vi "VisionLab_LHFind_Main.vi"() -> ()   [LabVIEW 2014]
uses:
  <vilib>/vision/Image Controls.llb/IMAQ Image.ctl
  <vilib>/userdefined/High Color/IMAQdx.ctl
  <vilib>/vision/driver/NI_Vision_Acquisition_Software.lvlib
panel:
  out "LH_Find":T1
  out "servo error out":errorcluster
  in  "Destination Point":cluster{"DestinationX":dbl, "DestinationY":dbl}={"DestinationX"=520.0, "DestinationY"=320.0}
  out "error out":errorcluster
  out "Live Input":T1(plugin-control)
  out "Running":bool
  in  "stop":bool
  out "FindLaser Out":T1(plugin-control)
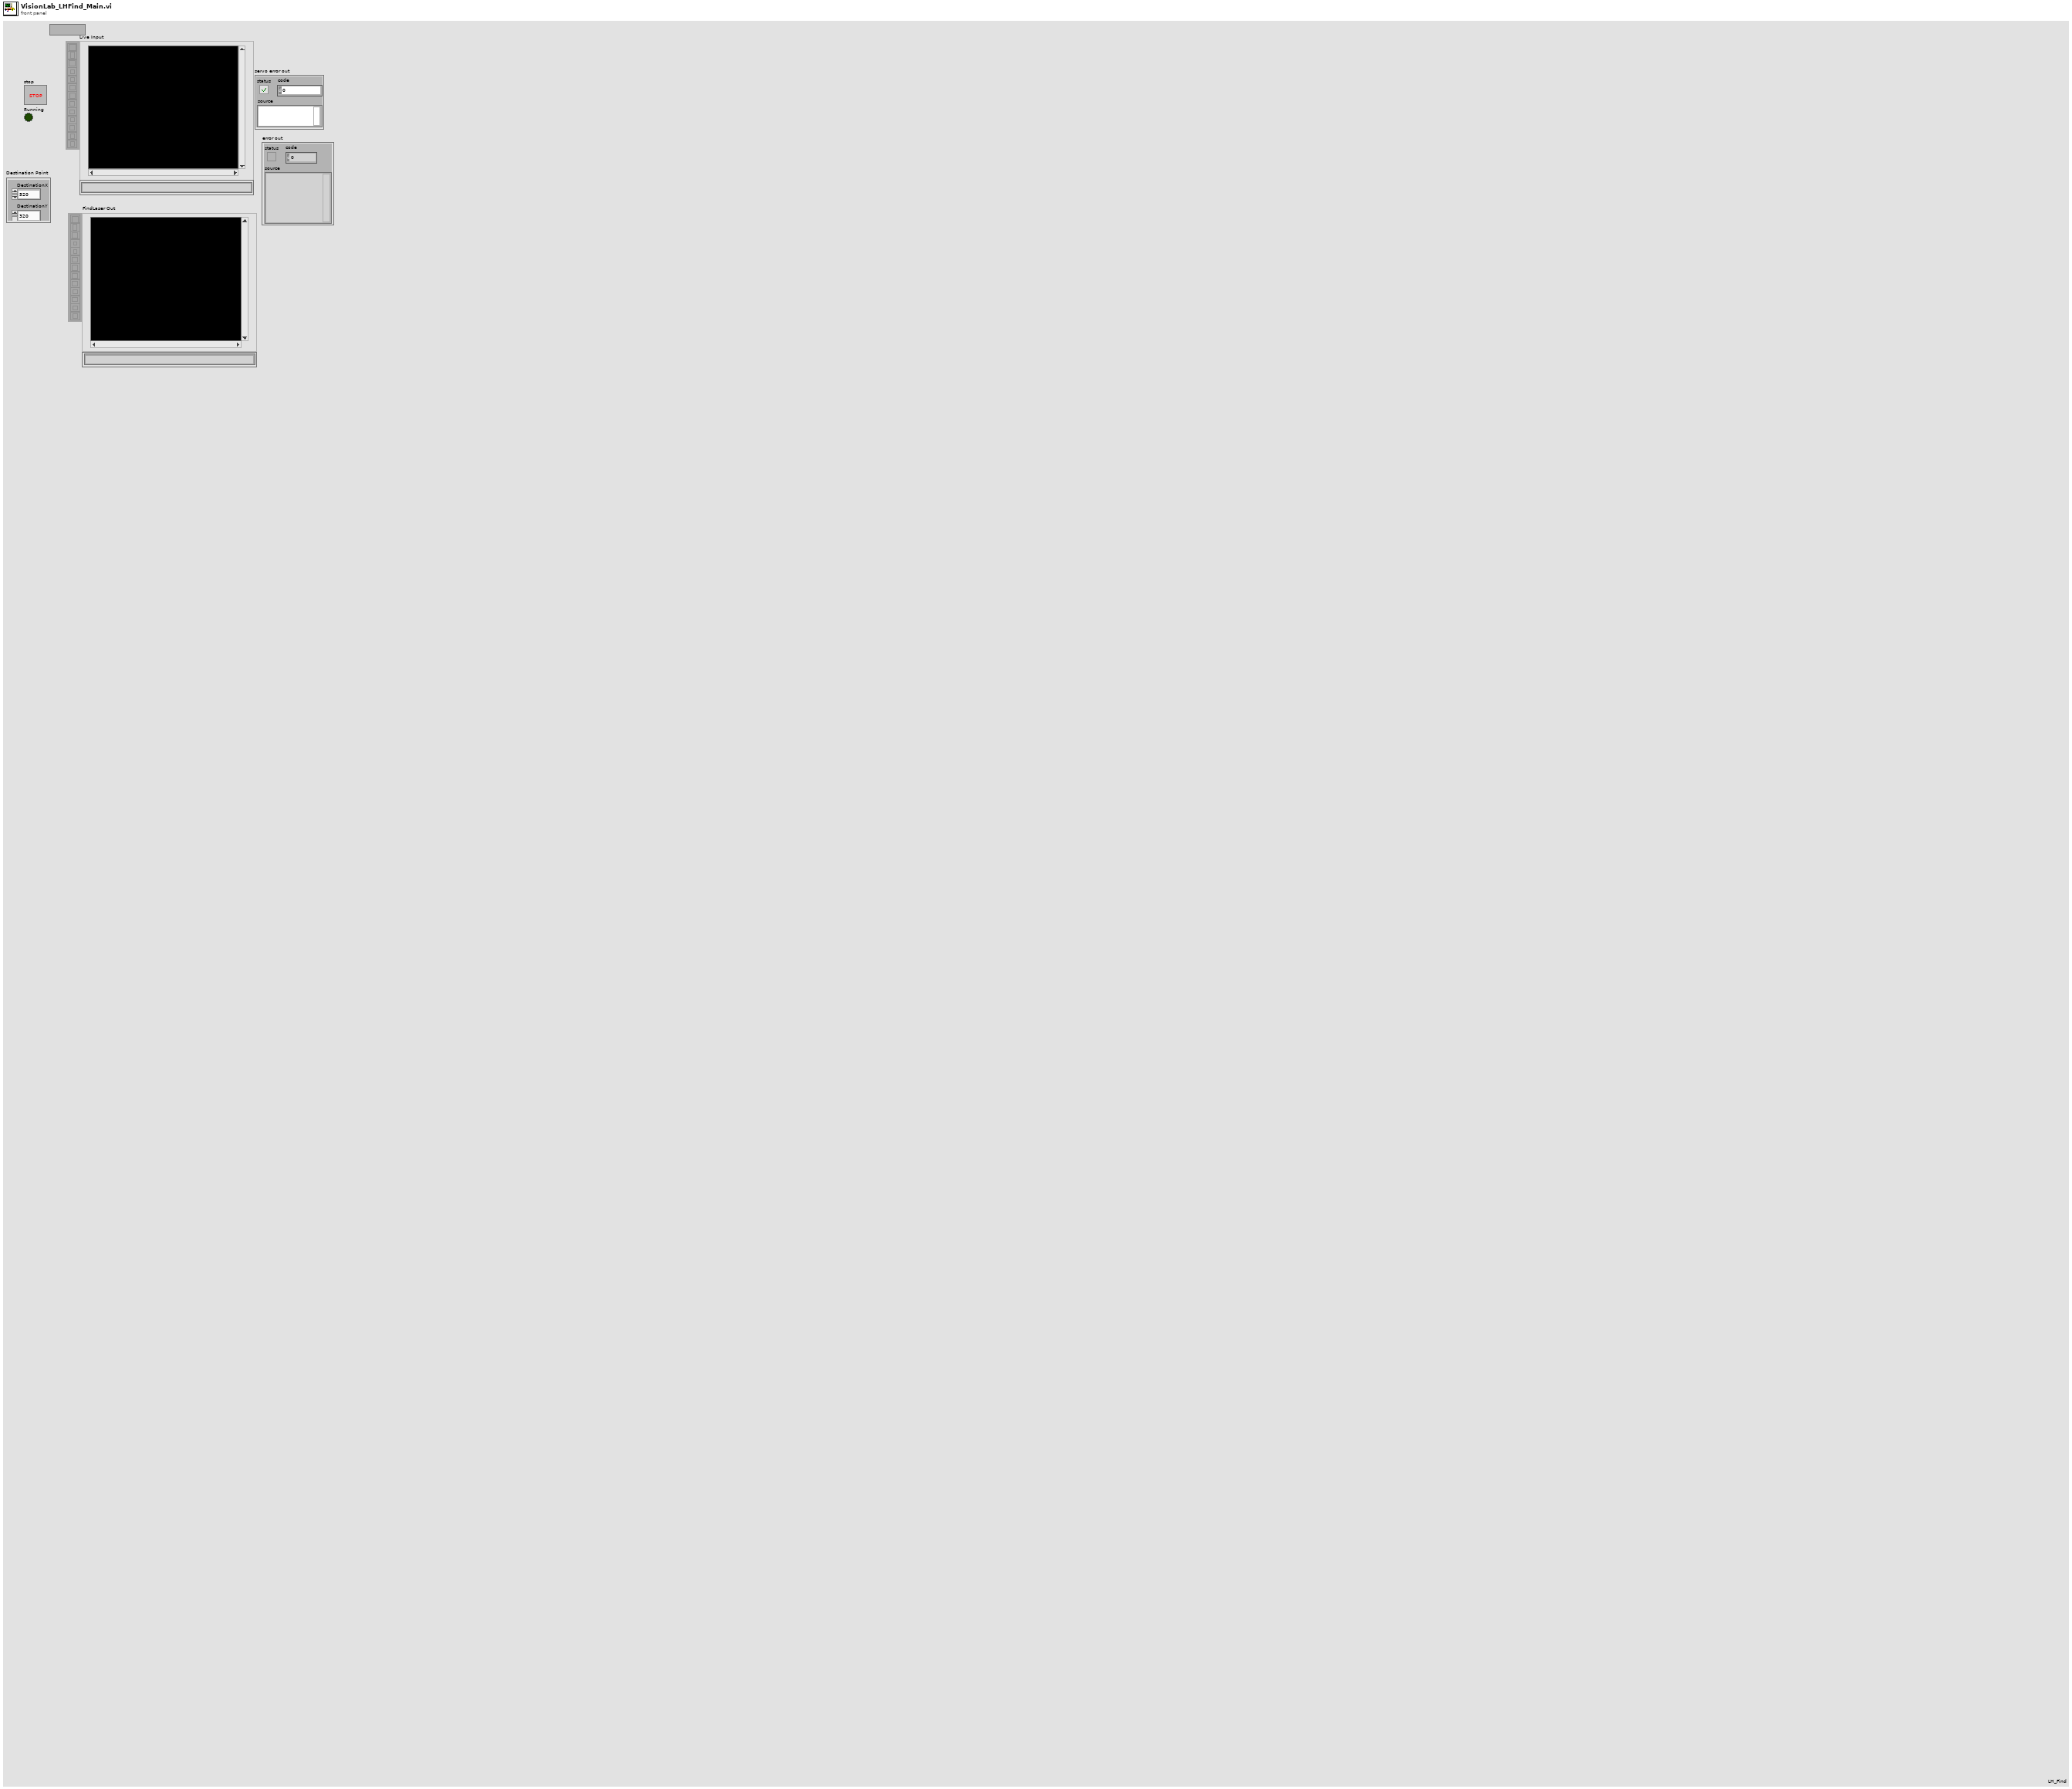
[diagram p1: front panel]
types:
  T1 = typedef "IMAQ Image.ctl" = refnum<image>
  T2 = typedef "IMAQdx.ctl" = refnum<k21>
  T3 = typedef "Image Type" = u32
  T4 = cluster{"Point1 (Pixels)":cluster{"X":sgl, "Y":sgl}, "Point2 (Pixels)":cluster{"X":sgl, "Y":sgl}, "Point1 (Real-World)":cluster{"X":sgl, "Y":sgl}, "Point2 (Real-World)":cluster{"X":sgl, "Y":sgl}, "Angle (Pixel)":dbl, "Angle (Real-World)":dbl, "Score":dbl, "Straightness":dbl, "Average SNR (db)":dbl, "Calibration Valid":bool}
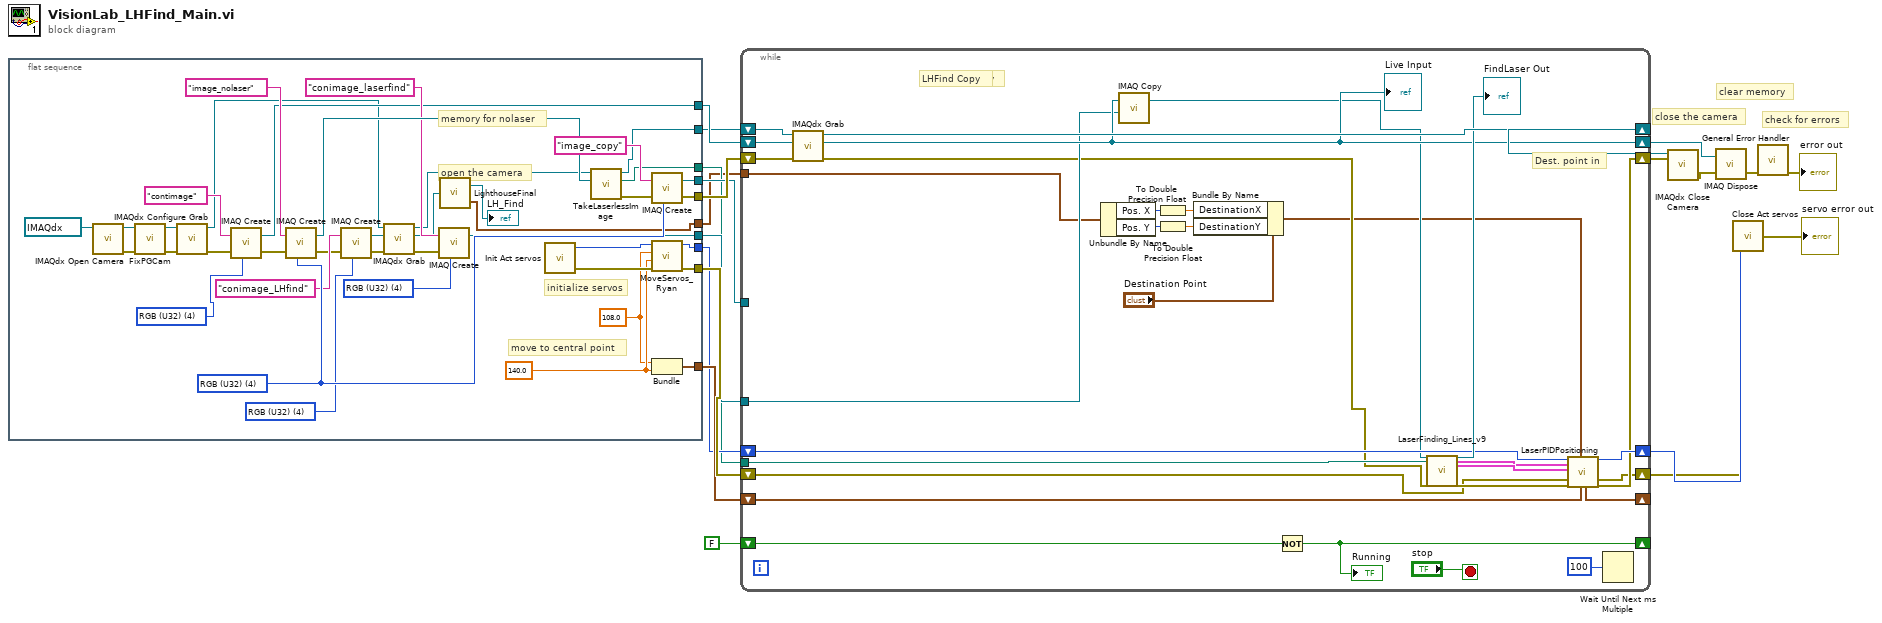
[diagram p0: block diagram]
diagram:
  # "check for errors"
  # "clear memory"
  # "close the camera"
  n1 = flat-sequence {
    tunnel: [w40] -> w20
    tunnel: [w31] -> w13
    tunnel: [w51] -> w6
    tunnel: [w49] -> w9
    tunnel: [w46] -> w7
    tunnel: [w39] -> w5
    tunnel: [w33] -> w4
    tunnel: [w32] -> w3
    tunnel: [w30] -> w2
    tunnel: [w21] -> w1
    frame #0 {
      w34 = T3 4 items=["Grayscale (U8)", "Grayscale (I16)", "Grayscale (SGL)", "Complex (CSG)", "RGB (U32)", "HSL (U32)", "RGB (U64)", "Grayscale (U16)"] ("Image Type")
      w37 = T3 4 items=["Grayscale (U8)", "Grayscale (I16)", "Grayscale (SGL)", "Complex (CSG)", "RGB (U32)", "HSL (U32)", "RGB (U64)", "Grayscale (U16)"] ("Image Type")
      w41 = T3 4 items=["Grayscale (U8)", "Grayscale (I16)", "Grayscale (SGL)", "Complex (CSG)", "RGB (U32)", "HSL (U32)", "RGB (U64)", "Grayscale (U16)"] ("Image Type")
      w47 = 108.0 ("Y pos")
      w48 = 140.0 ("X pos")
      w58 = T3 4 items=["Grayscale (U8)", "Grayscale (I16)", "Grayscale (SGL)", "Complex (CSG)", "RGB (U32)", "HSL (U32)", "RGB (U64)", "Grayscale (U16)"] ("Image Type")
      # "memory for nolaser"
      # "move to central point"
      # "initialize servos"
      # "open the camera"
      n2 = call <vilib>:"IMAQdx Open Camera.vi"("Session In"=T2 "cam1") -> ("error out"=w54:errorcluster, "Session Out"=w53:T2)  [unwired: 2 in, 7 out]
      n3 = call "FixPGCam.vi"("error in"=w54, "Session In"=w53) -> ("error out"=w56:errorcluster, "IMAQdx Session Out"=w55:T2)  [unwired: 8 in]
      n4 = call <vilib>:"IMAQdx Configure Grab.vi"("error in"=w56, "Session In"=w55) -> ("error out"=w57:errorcluster, "Session Out"=w25:T2)  [unwired: 8 out]
      n5 = call "IMAQ Create"("Image Name"="contimage", "Image Type"=w58, "error in (no error)"=w57) -> ("New Image"=w31:T1, "error out"=w45:errorcluster)  [unwired: 1 in, 1 out]
      n6 = call "IMAQ Create"("Image Name"="image_nolaser", "Image Type"=w41, "error in (no error)"=w45) -> ("New Image"=w43:T1, "error out"=w36:errorcluster)  [unwired: 1 in, 1 out]
      n7 = call "IMAQ Create"("Image Name"="conimage_LHfind", "Image Type"=w37, "error in (no error)"=w36) -> ("New Image"=w22:T1, "error out"=w27:errorcluster)  [unwired: 1 in, 1 out]
      n8 = call <vilib>:"IMAQdx Grab.vi"("error in"=w27, "Image In"=w22, "Session In"=w25) -> ("error out"=w26:errorcluster, "Image Out"=w23:T1, "Session Out"=w24:T2)  [unwired: 1 in, 5 out]
      n9 = call "IMAQ Create"("Image Name"="conimage_laserfind", "Image Type"=w34, "error in (no error)"=w26) -> ("New Image"=w33:T1)  [unwired: 1 in, 2 out]
      n10 = call "LighthouseFinal.vi"("Image In"=w23) -> ("Image Out"=→"LH_Find":T1, "output cluster"=w30:cluster{"Pos. X":i32, "Pos. Y":i32})
      n11 = call "Init Act servos.vi"() -> ("Device Out"=w52:i32, "error out"=w50:errorcluster)  [unwired: 1 in, 1 out]
      n12 = call "TakeLaserlessImage.vi"("Image In"=w43, "Session In"=w24) -> ("error out"=w28:errorcluster, "nolaser Filepath"=w32:path, "Session Out"=w21:T2)  [unwired: 7 in]
      n13 = call "IMAQ Create"("Image Name"="image_copy", "Image Type"=w41, "error in (no error)"=w28) -> ("New Image"=w39:T1, "error out"=w40:errorcluster)  [unwired: 2 in]
      n14 = call "MoveServos_Ryan.vi"("servo error in"=w50, "Y pos"=w48, "X pos"=w47, "Device In"=w52) -> ("servo error out"=w49:errorcluster, "Device Out"=w51:i32)  [unwired: 6 in]
      n15 = Bundle("Y pos"=w47, "X pos"=w48) -> (w46:cluster{"Y pos":dbl, "X pos":dbl})  [unwired: 1 in]
    }
  }
  n16 = while {
    shift-right: [w88] -> w19
    shift-left: w1 -> [w90]
    shift-right: [w72] -> w17
    shift-left: w13 -> [w83]
    shift-right: [w77] -> w11
    shift-left: w20 -> [w89]
    shift-right: [w86] -> _
    shift-left: FALSE -> [w87]
    shift-right: [w80] -> w12
    shift-left: w6 -> [w73]
    shift-right: [w79] -> _
    shift-left: w7 -> [w78]
    shift-right: [w74] -> w8
    shift-left: w9 -> [w75]
    tunnel: w5 -> [_]
    tunnel: w4 -> [w71]
    tunnel: w3 -> [w69]
    tunnel: w2 -> [w67]
    stop <- "stop" stop-if-true
    # "LaserFind Copy"
    # "LHFind Copy"
    # "Dest. point in"
    n17 = call <vilib>:"IMAQdx Grab.vi"("error in"=w89, "Image In"=w83, "Session In"=w90) -> ("error out"=w68:errorcluster, "Image Out"=w72:T1, "Session Out"=w88:T2)  [unwired: 1 in, 5 out]
    "Live Input" <- w72
    n18 = Unbundle By Name(w67) -> ("Pos. X"=w65:i32, "Pos. Y"=w64:i32)
    n19 = call "IMAQ Copy"("Image Dst"=w71, "Image Src"=w72) -> ("Image Dst Out"=w70:T1)  [unwired: 4 in, 1 out]
    n20 = To Double Precision Float(number=w65) -> (double precision float=w62:dbl)
    n21 = To Double Precision Float(number=w64) -> (double precision float=w63:dbl)
    n22 = Bundle By Name(cluster="Destination Point", "DestinationX"=w62, "DestinationY"=w63) -> (w61:cluster{"DestinationX":dbl, "DestinationY":dbl})
    n23 = Not(x=w87) -> (.not. x?=w86:bool)
    "Running" <- w86
    n24 = call "LaserFinding_Lines_v9.vi"("Image In"=w70, "File Path (Get Image without Laser)"=w69, "error in"=w68) -> ("Image Out"=→"FindLaser Out":T1, "Straight Edge (Find Vert. Edge)"=w81:T4, "Straight Edge (Find Horiz. Edge)"=w82:T4, "error out"=w76:errorcluster)  [unwired: 21 in]
    n25 = call "LaserPIDPositioning.vi"("Servo Device In"=w73, "Vertical Edge"=w81, "Horizontal Edge"=w82, "servo error in"=w75, "error in"=w76, "Destination Point"=w61, "Servo Angles In"=w78) -> ("Servo Angles Out"=w79:cluster{"Angle X":dbl, "Angle Y":dbl}, "Servo Device Out"=w80:i32, "servo error out"=w74:errorcluster, "error out"=w77:errorcluster)  [unwired: 9 in]
    n26 = Wait Until Next ms Multiple(millisecond multiple=u32 100 ("milliseconds to wait")) -> ()  [unwired: 1 out]
  }
  n27 = call <vilib>:"IMAQdx Close Camera.vi"("error in"=w11, "Session In"=w19) -> ("error out"=w18:errorcluster)  [unwired: 9 out]
  n28 = call "IMAQ Dispose"("Image"=w17, "error in (no error)"=w18) -> ("error out"=w16:errorcluster)  [unwired: 1 in, 3 out]
  n29 = call "Close Act servos.vi"("error in"=w8, "Device In"=w12) -> ("error out"=→"servo error out":errorcluster)
  n30 = call <vilib>:"General Error Handler.vi"("error in (no error)"=w16) -> ("error out"=→"error out":errorcluster)  [unwired: 2 in, 12 out]
